vi "LithographyObjects.vi"(8 "error in (no error)":errorcluster, 11 "AFM_Driver in":refnum<class "AFM_Driver.lvclass">) -> (0 "error out":errorcluster, 3 "AFM_Driver out":refnum<class "AFM_Driver.lvclass">)   [LabVIEW 2019, in "AFM_Driver.lvclass"]
uses:
  AFM_Driver.lvclass
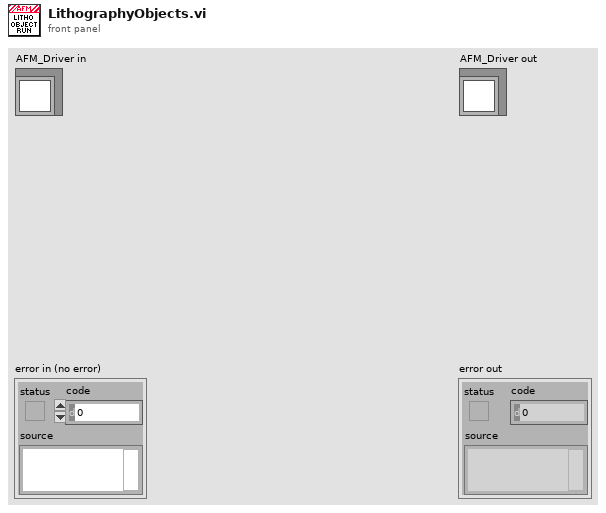
[diagram p1: front panel]
types:
  T1 = typedef "Relay-Box.lvclass/Resistor--enum.ctl" = enum16{"open", "discharge tip", "0 ohms", "100k ohm", "10M ohm", "1G ohm"}
  T2 = cluster{"Name":string, "Litho":cluster{"X":dbl, "Y":dbl, "Speed":dbl, "Voltage":dbl}[], "Set Resistance":T1, "Meta":variant}[]
  T3 = cluster{"X":dbl, "Y":dbl, "Speed":dbl, "Voltage":dbl}[]
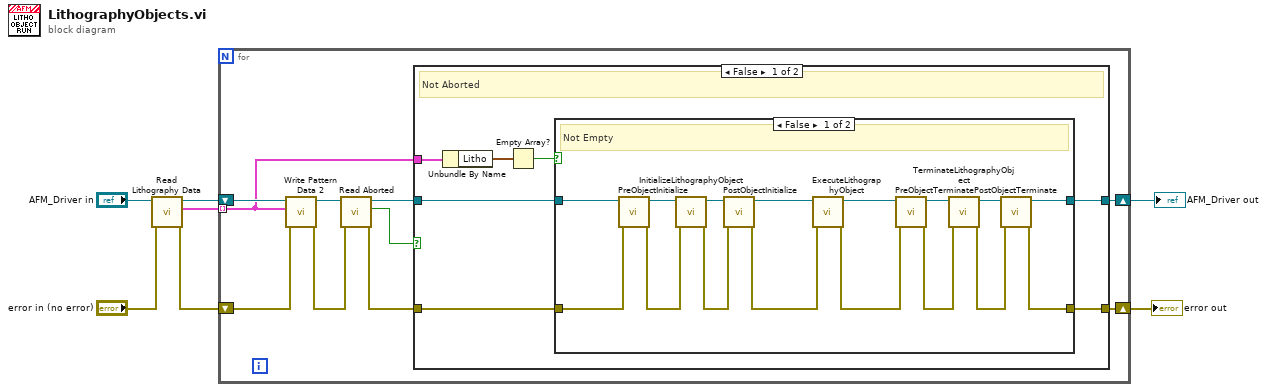
[diagram p0: block diagram]
diagram:
  n1 = call-dynamic "Read Lithography Data.vi"("error in (no error)"="error in (no error)", "AFM_Driver in"="AFM_Driver in") -> ("error out"=w1:errorcluster, "Lithography Data"=w3:T2, "AFM_Driver out"=w4:refnum<class "AFM_Driver.lvclass">)  [unwired: 7 in]
  n2 = for {
    shift-right: [w16] -> w6
    shift-left: w4 -> [w15]
    shift-right: [w17] -> w7
    shift-left: w1 -> [w14]
    tunnel: w3 -> [w13] mode=indexing
    n3 = call-dynamic "Write Pattern Data 2.vi"("error in (no error)"=w14, "Pattern Data"=w13, "AFM_Driver in"=w15) -> ("error out"=w10:errorcluster, "AFM_Driver out"=w12:refnum<class "AFM_Driver.lvclass">)  [unwired: 7 in]
    n4 = call "Read Aborted.vi"("error in (no error)"=w10, "AFM_Driver in"=w12) -> ("error out"=w9:errorcluster, "Aborted?"=w8:bool, "AFM_Driver out"=w11:refnum<class "AFM_Driver.lvclass">)  [unwired: 7 in]
    n5 = case shown="False" w8 {
      tunnel: w9 -> [w20 w44]
      tunnel: [w24 w44] -> w17
      tunnel: w11 -> [w21 w43]
      tunnel: [w22 w43] -> w16
      tunnel: w13 -> [w19 _]
      frame False {
        # "Not Aborted"
        n6 = Unbundle By Name(w19) -> ("Litho"=w18:T3)
        n7 = Empty Array?(array=w18) -> (empty?=w23:bool)
        n8 = case shown="False" w23 {
          tunnel: w20 -> [w26 w42]
          tunnel: [w25 w42] -> w24
          tunnel: [w28 w41] -> w22
          tunnel: w21 -> [w27 w41]
          frame False {
            # "Not Empty"
            n9 = call-dynamic "PreObjectInitialize.vi"("error in (no error)"=w26, "AFM.Asylum in"=w27) -> ("error out"=w39:errorcluster, "AFM.Asylum out"=w40:refnum<class "AFM_Driver.lvclass">)  [unwired: 8 in]
            n10 = call-dynamic "InitializeLithographyObject.vi"("error in (no error)"=w39, "AFM_Driver in"=w40) -> ("error out"=w37:errorcluster, "AFM_Driver out"=w38:refnum<class "AFM_Driver.lvclass">)  [unwired: 8 in]
            n11 = call-dynamic "PostObjectInitialize.vi"("error in (no error)"=w37, "AFM_Driver in"=w38) -> ("error out"=w35:errorcluster, "AFM_Driver out"=w36:refnum<class "AFM_Driver.lvclass">)  [unwired: 8 in]
            n12 = call-dynamic "ExecuteLithographyObject.vi"("error in (no error)"=w35, "AFM_Driver in"=w36) -> ("error out"=w33:errorcluster, "AFM_Driver out"=w34:refnum<class "AFM_Driver.lvclass">)  [unwired: 8 in]
            n13 = call-dynamic "PreObjectTerminate.vi"("error in (no error)"=w33, "AFM_Driver in"=w34) -> ("error out"=w31:errorcluster, "AFM_Driver out"=w32:refnum<class "AFM_Driver.lvclass">)  [unwired: 8 in]
            n14 = call-dynamic "TerminateLithographyObject.vi"("error in (no error)"=w31, "AFM_Driver in"=w32) -> ("error out"=w29:errorcluster, "AFM_Driver out"=w30:refnum<class "AFM_Driver.lvclass">)  [unwired: 8 in]
            n15 = call-dynamic "PostObjectTerminate.vi"("error in (no error)"=w29, "AFM_Driver in"=w30) -> ("error out"=w25:errorcluster, "AFM_Driver out"=w28:refnum<class "AFM_Driver.lvclass">)  [unwired: 8 in]
          }
          frame True {
          }
        }
      }
      frame True {
      }
    }
  }
  "error out" <- w7
  "AFM_Driver out" <- w6
